vi "fgt get ttl channels Info.vi"(8 "error in (no error)":errorcluster) -> (0 "error out":errorcluster, 3 "TTL channels info":T1[](array[typedef]))   [LabVIEW 2020, in "fgt_SDK.lvlib"]
doc: "Retrieve information about each initialized TTL channel. This function is useful in order to get channels order, controller, unique ID and InstrType.\nTTL channels are only available for LineUP Series, 2 ports for each connected Link"
uses:
  fgt_SDK.lvlib
  TypeDefs/fgt_CHANNEL_INFO.ctl
  TypeDefs/fgt_INSTRUMENT_TYPE.ctl
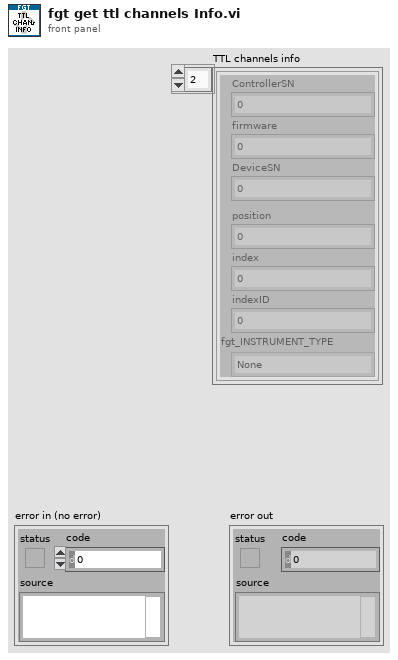
[diagram p1: front panel]
types:
  T1 = typedef "fgt_SDK.lvlib/fgt_CHANNEL_INFO.ctl" = cluster{"ControllerSN":u16, "firmware":u16, "DeviceSN":u16, "position":u32, "index":u32, "indexID":u32, "fgt_INSTRUMENT_TYPE":T2}
  T2 = typedef "fgt_SDK.lvlib/fgt_INSTRUMENT_TYPE.ctl" = enum32{"None", "MFCS", "MFCS_EZ", "FRP", "LineUP", "IPS"}
  T3 = cluster{"ControllerSN":u16, "firmware":u16, "DeviceSN":u16, "Padding":u16, "position":u32, "index":u32, "indexID":u32, "fgt_INSTRUMENT_TYPE":T2}
  T4 = cluster{"ControllerSN":u16, "firmware":u16, "DeviceSN":u16, "Padding":u16, "position":u32, "index":u32, "indexID":u32, "fgt_INSTRUMENT_TYPE":T2}[]
  T5 = typedef "fgt_SDK.lvlib/fgt_STATUS_INFO.ctl" = cluster{"InstrType":T2, "instrSN":u16, "errorCode":u8, "infoCode":u8, "detail":string}
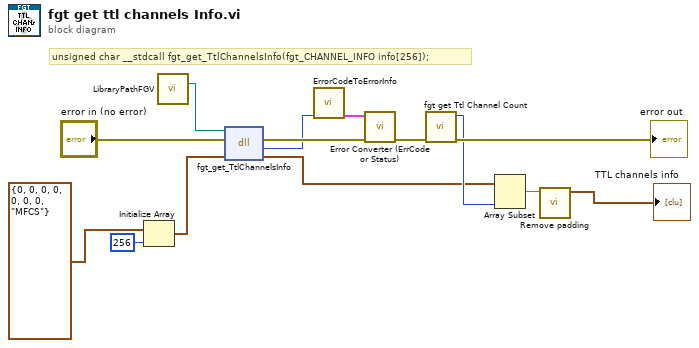
[diagram p0: block diagram]
diagram:
  # "unsigned char __stdcall fgt_get_TtlChannelsInfo(fgt_CHANNEL_INFO info[256]);"
  n1 = Initialize Array(T3 {"ControllerSN"=0, "firmware"=0, "DeviceSN"=0, "Padding"=0, "position"=0, "index"=0, "indexID"=0, "fgt_INSTRUMENT_TYPE"=enum."MFCS"} ("fgt_CHANNEL_INFO"), 256 ("dimension size")) -> (w9:T4)
  n2 = call "LibraryPathFGV.vi"() -> ("Path Out"=w1:path)  [unwired: 14 in, 1 out]
  n3 = dll-call lib="C:/Workspace/fgt-SDK/LabVIEW/dlls/fgt_SDK_*.*" fn="fgt_get_TtlChannelsInfo"(path in=w1, error in="error in (no error)", "info"=w9) -> (error out=w13:errorcluster, "return type"=w12:u8, "info"=w5:T4)  [unwired: 1 in, 1 out]
  n4 = call "ErrorCodeToErrorInfo.vi"("return type"=w12) -> ("StatusInfo"=w11:T5)  [unwired: 10 in]
  n5 = call "Error Converter (ErrCode or Status).vi"("error in (no error)"=w13, "StatusInfo"=w11) -> ("error out"=w8:errorcluster)  [unwired: 9 in]
  n6 = call "fgt get Ttl Channel Count.vi"("error in (no error)"=w8) -> ("error out"=→"error out":errorcluster, "nbTtlChan out"=w6:u32)  [unwired: 9 in]
  n7 = Array Subset(array=w5, length=w6) -> (w3:T4)  [unwired: 1 in]
  n8 = call "Remove padding.vi"("Array in"=w3) -> ("Array out"=→"TTL channels info":T1[])  [unwired: 10 in]
